vi "WFAppendD.vi"(0 "Waveform In":digitalwaveform(waveform)={"t0"=timestamp(0 s since 1904-01-01), "dt"=1.0, "Y"={"transitions"=[], "data"=[]}}, 1 "Waveform In 2":digitalwaveform(waveform)={"t0"=timestamp(0 s since 1904-01-01), "dt"=1.0, "Y"={"transitions"=[], "data"=[]}}, 2 "Waveform In 3":digitalwaveform(waveform)={"t0"=timestamp(0 s since 1904-01-01), "dt"=1.0, "Y"={"transitions"=[], "data"=[]}}, 3 "Waveform In 4":digitalwaveform(waveform)={"t0"=timestamp(0 s since 1904-01-01), "dt"=1.0, "Y"={"transitions"=[], "data"=[]}}, 4 "Waveform In 5":digitalwaveform(waveform)={"t0"=timestamp(0 s since 1904-01-01), "dt"=1.0, "Y"={"transitions"=[], "data"=[]}}, 5 "error in (no error)":errorcluster) -> (14 "Waveform Out":digitalwaveform(waveform)={"t0"=timestamp(0 s since 1904-01-01), "dt"=1.0, "Y"={"transitions"=[], "data"=[]}}, 19 "error out":errorcluster)   [LabVIEW 2013]
uses:
  WFAppend2D.vi
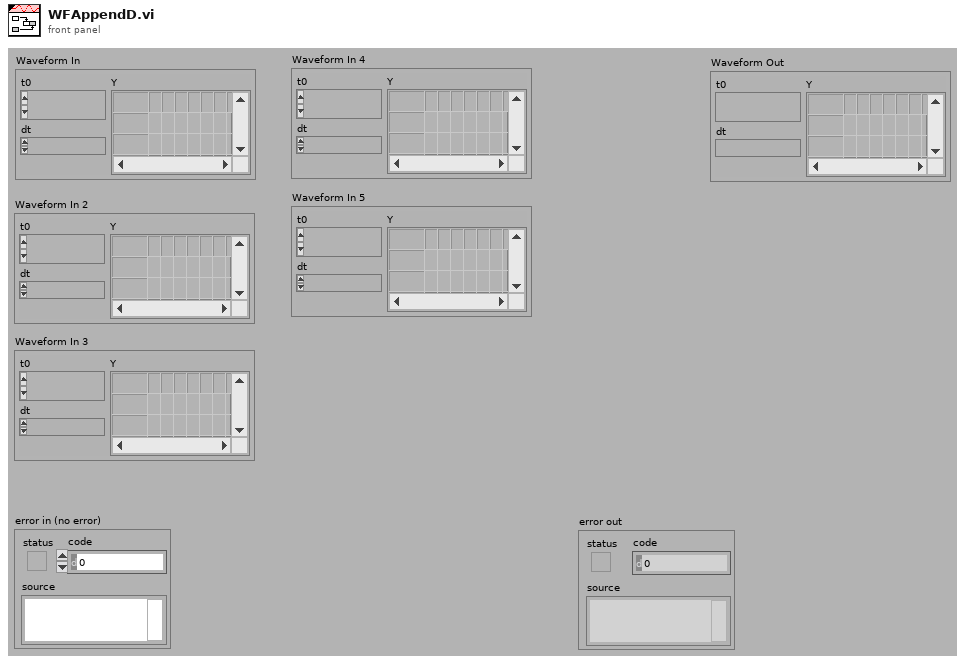
[diagram p1: front panel]
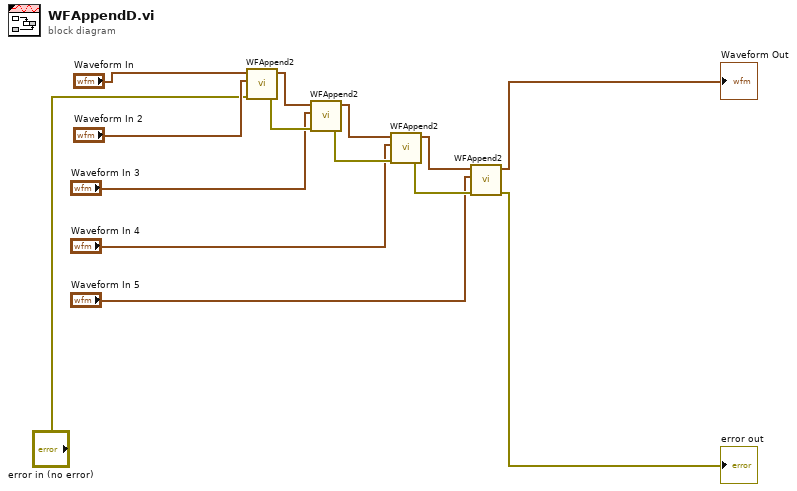
[diagram p0: block diagram]
diagram:
  n1 = call-poly "WFAppend2.vi"("error in (no error)"="error in (no error)", "Waveform In 2"="Waveform In 2", "Waveform In"="Waveform In") -> ("error out"=w13:errorcluster, "Waveform Out"=w14:digitalwaveform)  [unwired: 3 in]
  n2 = call-poly "WFAppend2.vi"("error in (no error)"=w13, "Waveform In 2"="Waveform In 3", "Waveform In"=w14) -> ("error out"=w11:errorcluster, "Waveform Out"=w12:digitalwaveform)  [unwired: 3 in]
  n3 = call-poly "WFAppend2.vi"("error in (no error)"=w11, "Waveform In 2"="Waveform In 4", "Waveform In"=w12) -> ("error out"=w9:errorcluster, "Waveform Out"=w10:digitalwaveform)  [unwired: 3 in]
  n4 = call-poly "WFAppend2.vi"("error in (no error)"=w9, "Waveform In 2"="Waveform In 5", "Waveform In"=w10) -> ("error out"=→"error out":errorcluster, "Waveform Out"=→"Waveform Out":digitalwaveform)  [unwired: 3 in]
